vi "midpoint.vi"(10 "UTM Location 2":T1 {"North" format="%#_10f"; "East" format="%#_8f"}, 11 "UTM Location":T1 {"North" format="%#_10f"; "East" format="%#_8f"}) -> (2 "Distance":dbl, 3 "UTM Location 3":T1 {"North" format="%#_10f"; "East" format="%#_8f"})   [LabVIEW 2013]
doc: "Finds the midpoint between two UTM coordinates and returns it in UTM.\n\nDoes not take into account UTM zones or hemispheres."
uses:
  Data/TypeDefs/UTM Location.ctl
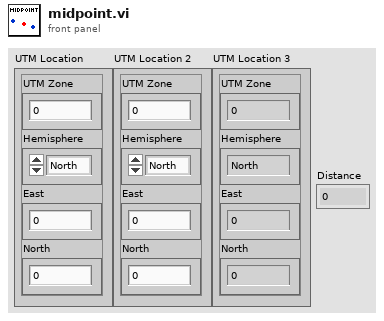
[diagram p1: front panel]
types:
  T1 = typedef "UTM Location.ctl" = cluster{"UTM Zone":dbl, "Hemisphere":enum16{"North", "South"}, "East":dbl, "North":dbl}
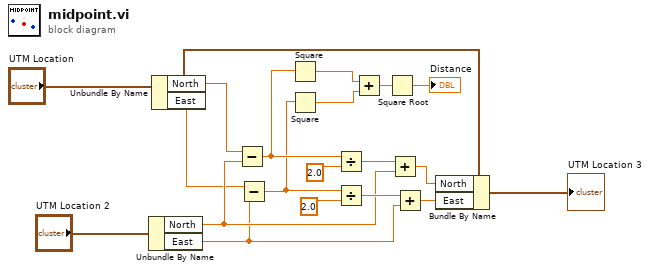
[diagram p0: block diagram]
diagram:
  n1 = Unbundle By Name("UTM Location 2") -> ("North"=w15:dbl, "East"=w14:dbl)
  n2 = Unbundle By Name("UTM Location") -> ("North"=w11:dbl, "East"=w10:dbl)
  n3 = Subtract(x=w11, y=w15) -> (x-y=w6:dbl)
  n4 = Subtract(x=w10, y=w14) -> (x-y=w5:dbl)
  n5 = Square(x=w6) -> (x^2=w8:dbl)
  n6 = Square(x=w5) -> (x^2=w9:dbl)
  n7 = Divide(x=w6, y=2.0) -> (x/y=w16:dbl)
  n8 = Divide(x=w5, y=2.0) -> (x/y=w17:dbl)
  n9 = Add(x=w8, y=w9) -> (x+y=w7:dbl)
  n10 = Square Root(x=w7) -> (sqrt(x)=→"Distance":dbl)
  n11 = Add(x=w16, y=w15) -> (x+y=w12:dbl)
  n12 = Add(x=w17, y=w14) -> (x+y=w13:dbl)
  n13 = Bundle By Name(cluster="UTM Location", "North"=w12, "East"=w13) -> (→"UTM Location 3":T1)
